vi "Calc Profile Data Structure Size.vi"(9 "Profile Data Point":u16, 11 "Profile Cnt":u8=1) -> (1 "Profile Size(DWORD)":u32, 3 "Profile Size(Byte)":u32)   [LabVIEW 2015, in "KEYENCE LJ-X8000A.lvlib"]
uses:
  KEYENCE LJ-X8000A.lvlib
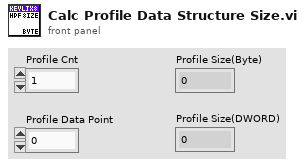
[diagram p1: front panel]
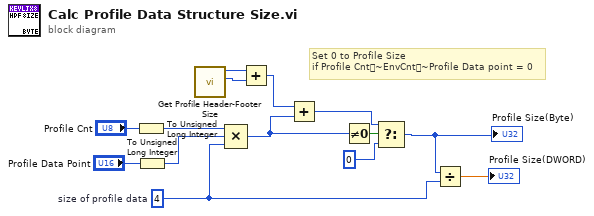
[diagram p0: block diagram]
diagram:
  w2 = u32 4  # size of profile data
  # "Set 0 to Profile Size\nif Profile Cnt~EnvCnt~Profile Data point = 0"
  n1 = To Unsigned Long Integer(number="Profile Cnt") -> (unsigned 32bit integer=w5:u32)
  n2 = To Unsigned Long Integer(number="Profile Data Point") -> (unsigned 32bit integer=w12:u32)
  n3 = call "Get Profile Header-Footer Size.vi"() -> ("Footer Size(Byte)"=w4:u32, "Header Size(Byte)"=w11:u32)  [unwired: 8 in, 2 out]
  n4 = Compound Arithmetic op=MULTIPLY(w5, w12, w2) -> (w8:u32)
  n5 = Add(x=w11, y=w4) -> (x+y=w10:u32)
  n6 = Add(x=w10, y=w8) -> (x+y=w7:u32)
  n7 = Not Equal To 0?(x=w8) -> (x != 0?=w9:bool)
  n8 = Select(t=w7, s=w9, f=u32 0) -> (s? t:f=w3:u32)
  "Profile Size(Byte)" <- w3
  n9 = Divide(x=w3, y=w2) -> (x/y=→"Profile Size(DWORD)":dbl)
